vi "Pretty Print Level.vi"(8 "error in (no error)":errorcluster, 10 "Action":enum16{"Increment", "Decrement", "Get", "Reset"}(ring)) -> (0 "error out":errorcluster, 2 "Numeric":i32)   [LabVIEW 2016, in "JSON Helper.lvclass"]
doc: "FGV used to determine the current indentation when pretty printing."
uses:
  JSON Data Classes/JSON Helper/JSON Helper.lvclass
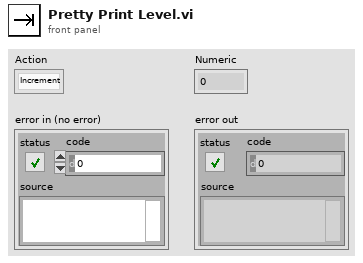
[diagram p1: front panel]
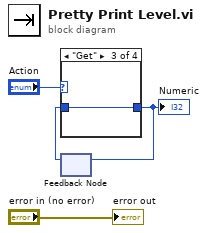
[diagram p0: block diagram]
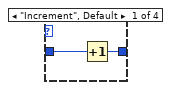
[diagram p2: hidden frame]
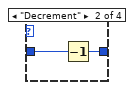
[diagram p3: hidden frame]
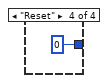
[diagram p4: hidden frame]
diagram:
  n1 = feedback #1() -> (w2:i32)  [unwired: 1 in]
  n2 = case shown="\"Get\"" "Action" {
    tunnel: [w5 w7 w9 0] -> w3
    tunnel: w2 -> [w6 w8 w9 _]
    frame "Increment", Default {
      n3 = Increment(x=w6) -> (x+1=w5:i32)
    }
    frame "Decrement" {
      n4 = Decrement(x=w8) -> (x-1=w7:i32)
    }
    frame "Get" {
    }
    frame "Reset" {
    }
  }
  "Numeric" <- w3
  n5 = feedback-in #1(w3) -> ()
  "error out" <- "error in (no error)"
